vi "sleepGyro.vi"(0 "enable":bool) -> ()   [LabVIEW 2016]
uses:
  testing/HawaiiTest1/modular_imu_vis/imuSubVIs/#defines.ctl
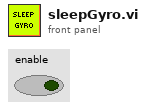
[diagram p1: front panel]
types:
  T1 = typedef "#defines.ctl" = i16
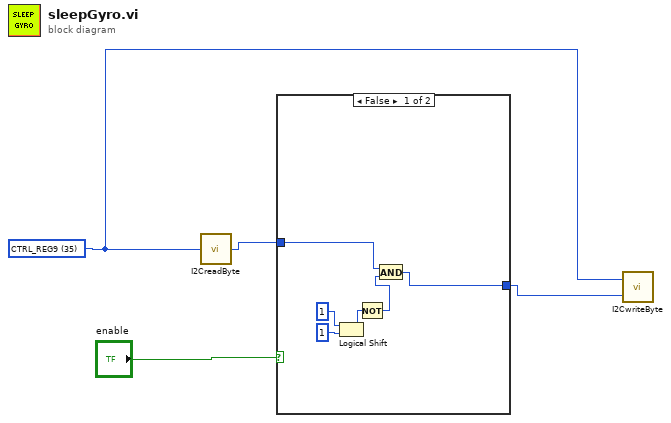
[diagram p0: block diagram]
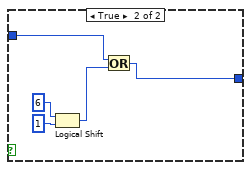
[diagram p2: hidden frame]
diagram:
  w1 = T1 35 items=["CTRL_REG9"=35, "STATUS_REG_1"=39, "OUT_X_L_XL"=40, "FIFO_CTRL"=46, "FIFO_SRC"=47, "CTRL_REG4"=30, "OUT_X_L_G"=24, "OUT_TEMP_L"=21, "INT_GEN_SRC_G"=20, "ORIENT_CFG_G"=19, "CTRL_REG3_G"=18, "CTRL_REG2_G"=17, "CTRL_REG1_G"=16, "WHO_AM_I_XG"=15] ("Ring")
  n1 = call "I2CreadByte.vi"("subAddress"=w1) -> ("data"=w3:u8)
  n2 = case shown="False" "enable" {
    tunnel: w3 -> [w8 w12]
    tunnel: [w5 w11] -> w2
    frame False {
      n3 = Logical Shift(y=i16 1, x=i16 1) -> (x << y=w7:i16)
      n4 = Not(x=w7) -> (.not. x?=w6:i16)
      n5 = And(x=w8, y=w6) -> (x .and. y?=w5:i16)
    }
    frame True {
      n6 = Logical Shift(y=i16 6, x=i16 1) -> (x << y=w13:i16)
      n7 = Or(x=w12, y=w13) -> (x .or. y?=w11:i16)
    }
  }
  n8 = call "I2CwriteByte.vi"("data"=w2, "subAddress"=w1) -> ()  [unwired: 1 in]
